vi "Read Number of Jobs.vi"(8 "error in (no error)":errorcluster, 11 "OSSP_Problem in":refnum<class "OSSP_Problem.lvclass">) -> (0 "error out":errorcluster, 2 "Number of Jobs":i32, 3 "OSSP_Problem out":refnum<class "OSSP_Problem.lvclass">)   [LabVIEW 2013, in "OSSP_Problem.lvclass"]
uses:
  OSSP_Problem.lvclass
  OSSP_Problem.lvclass/OSSP_Problem.ctl
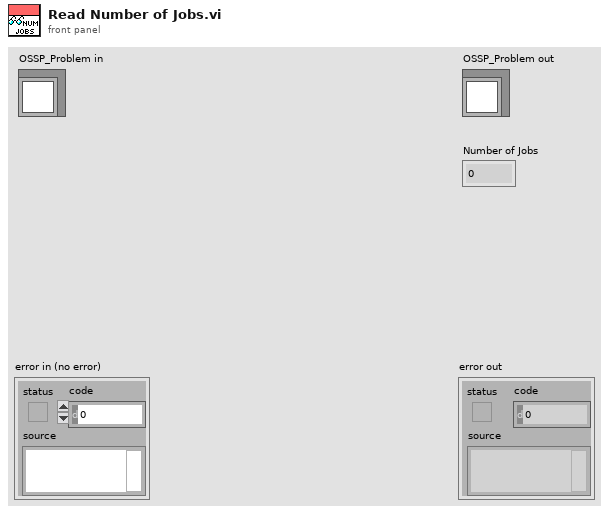
[diagram p1: front panel]
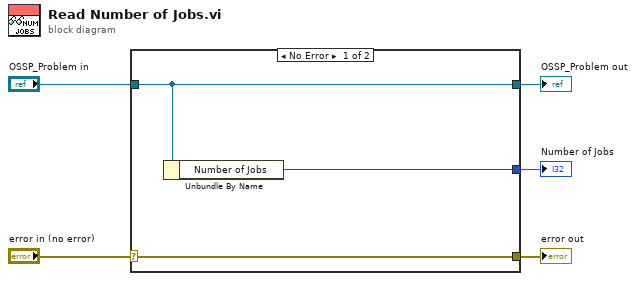
[diagram p0: block diagram]
diagram:
  n1 = case shown="No Error" "error in (no error)" {
    selector: "error in (no error)" -> [w8 w9]
    tunnel: [w8 w9] -> w4
    tunnel: [w7 w10] -> w2
    tunnel: "OSSP_Problem in" -> [w7 w10]
    tunnel: [w6 _] -> w1
    frame No Error {
      n2 = Unbundle By Name(w7) -> ("Number of Jobs"=w6:i32)
    }
    frame Error {
    }
  }
  "error out" <- w4
  "OSSP_Problem out" <- w2
  "Number of Jobs" <- w1
